vi "Get Attributes.vi"(8 "error in (no error)":errorcluster, 11 "GetTypeAttributesVisitor.lvclass in":refnum<class "GetTypeAttributesVisitor.lvclass">) -> (0 "error out":errorcluster, 2 "Attributes":T1[](array[typedef]), 3 "GetTypeAttributesVisitor.lvclass out":refnum<class "GetTypeAttributesVisitor.lvclass">)   [LabVIEW 2020, in "Web Service Description.lvlib" / "GetTypeAttributesVisitor.lvclass"]
uses:
  <vilib>/AppBuilder/Engine/WebServiceDescription/GetTypeAttributesVisitor/GetTypeAttributesVisitor.lvclass
  <vilib>/AppBuilder/Engine/WebServiceDescription/XMLGen/ValuePair.ctl
  <vilib>/AppBuilder/Engine/WebServiceDescription/GetTypeAttributesVisitor/GetTypeAttributesVisitor.lvclass/GetTypeAttributesVisitor.ctl
  <vilib>/AppBuilder/Engine/WebServiceDescription/XMLGen/XMLGen.lvlib
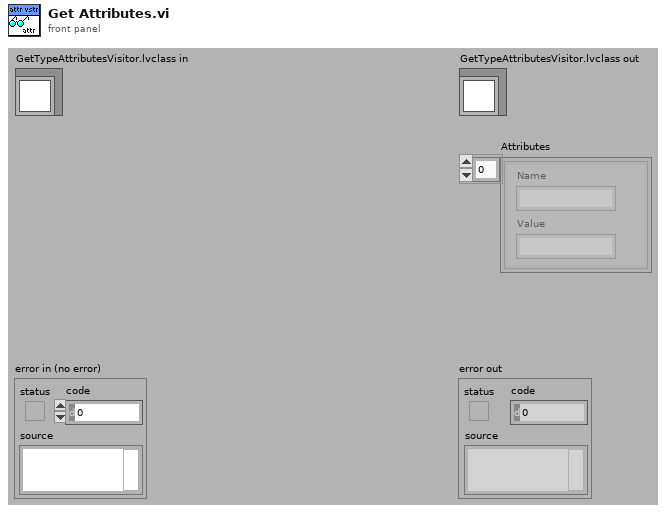
[diagram p1: front panel]
types:
  T1 = typedef "XMLGen.lvlib/ValuePair.ctl" = cluster{"Name":string, "Value":string}
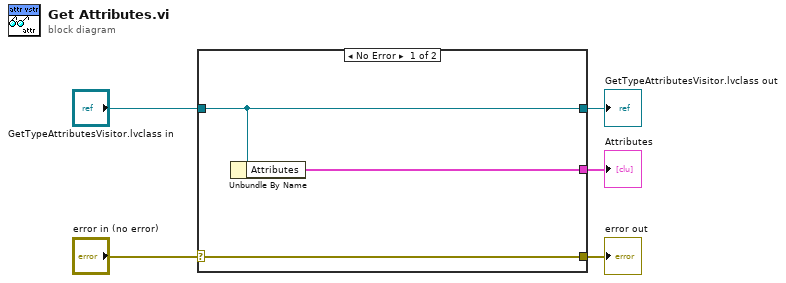
[diagram p0: block diagram]
diagram:
  n1 = case shown="No Error" "error in (no error)" {
    selector: "error in (no error)" -> [w8 w9]
    tunnel: [w8 w9] -> w4
    tunnel: [w7 w10] -> w2
    tunnel: "GetTypeAttributesVisitor.lvclass in" -> [w7 w10]
    tunnel: [w6 _] -> w1
    frame No Error {
      n2 = Unbundle By Name(w7) -> ("Attributes"=w6:T1[])
    }
    frame Error {
    }
  }
  "error out" <- w4
  "GetTypeAttributesVisitor.lvclass out" <- w2
  "Attributes" <- w1
